vi "Generate Ringdowns.vi"(0 "Ramp Pattern":dbl[](array[numeric]), 1 "Exp Data":cluster{"A":dbl, "B":dbl, "tau":dbl}[](array[cluster]), 5 "error in":errorcluster) -> (14 "RD Data Out":dbl[][](array[numeric]), 19 "error out":errorcluster)   [LabVIEW 2014]
uses:
  General/Math/Fit Exponential Class/Fit Exponential.lvclass
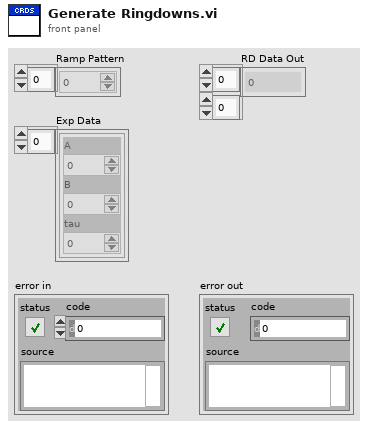
[diagram p1: front panel]
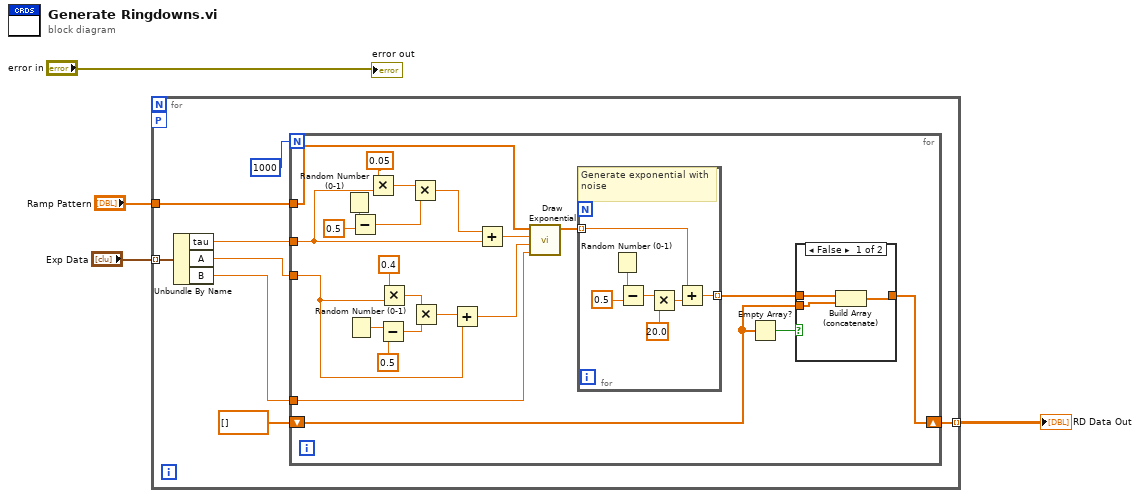
[diagram p0: block diagram]
diagram:
  n1 = for {
    tunnel: "Ramp Pattern" -> [w12]
    tunnel: [w9] -> w3 mode=indexing
    workers-P: _ -> [_]
    tunnel: "Exp Data" -> [w8] mode=indexing
    n2 = Unbundle By Name(w8) -> ("tau"=w6:dbl, "A"=w7:dbl, "B"=w5:dbl)
    n3 = for {
      N: 1000 -> [_]
      tunnel: w12 -> [w35]
      shift-right: [w31] -> w9
      shift-left: dbl[] [] -> [w30]
      tunnel: w6 -> [w15]
      tunnel: w7 -> [w14]
      tunnel: w5 -> [w13]
      n4 = Random Number (0-1)() -> (number: 0 to 1=w28:dbl)
      n5 = Random Number (0-1)() -> (number: 0 to 1=w19:dbl)
      n6 = Subtract(x=w28, y=0.5) -> (x-y=w25:dbl)
      n7 = Multiply(x=0.05 ("y"), y=w15) -> (x*y=w26:dbl)
      n8 = Subtract(x=w19, y=0.5) -> (x-y=w18:dbl)
      n9 = Multiply(x=0.4 ("y"), y=w14) -> (x*y=w21:dbl)
      n10 = Multiply(x=w26, y=w25) -> (x*y=w24:dbl)
      n11 = Multiply(x=w21, y=w18) -> (x*y=w17:dbl)
      n12 = Add(x=w17, y=w14) -> (x+y=w16:dbl)
      n13 = Add(x=w24, y=w15) -> (x+y=w23:dbl)
      n14 = call "Draw Exponential.vi"("B"=w13, "A"=w16, "tau"=w23, "time"=w35) -> ("ExponentialOut"=w34:dbl[])  [unwired: 7 in]
      n15 = for {
        tunnel: w34 -> [w41] mode=indexing
        tunnel: [w40] -> w32 mode=indexing
        # "Generate exponential with noise"
        n16 = Random Number (0-1)() -> (number: 0 to 1=w46:dbl)
        n17 = Subtract(x=w46, y=0.5) -> (x-y=w44:dbl)
        n18 = Multiply(x=w44, y=20.0) -> (x*y=w42:dbl)
        n19 = Add(x=w41, y=w42) -> (x+y=w40:dbl)
      }
      n20 = Empty Array?(array=w30) -> (empty?=w33:bool)
      n21 = case shown="False" w33 {
        tunnel: w32 -> [w38 w39]
        tunnel: [w36 w39] -> w31
        tunnel: w30 -> [w37 _]
        frame False {
          n22 = Build Array (concatenate)(w38, w37) -> (w36:dbl[])
        }
        frame True {
        }
      }
    }
  }
  "RD Data Out" <- w3
  "error out" <- "error in"
